vi "Find Item Locations by Path.vi"(5 "Insertion point if not found":bool, 6 "Only return first found":bool, 7 "Path":string, 8 "error in (no error)":errorcluster, 10 "Object Offset":i32, 11 "JSON":string) -> (0 "error out":errorcluster, 1 "Items":T1[](array[typedef]))   [LabVIEW 2017, in "JSONtext.lvlib"]
uses:
  JSONtext.lvlib
  Parsing/Found Items.ctl
  Parsing/Parsing State.ctl
  <vilib>/JDP Science/JDP Science Common Utilities/Trim Whitespace__JDP.vi
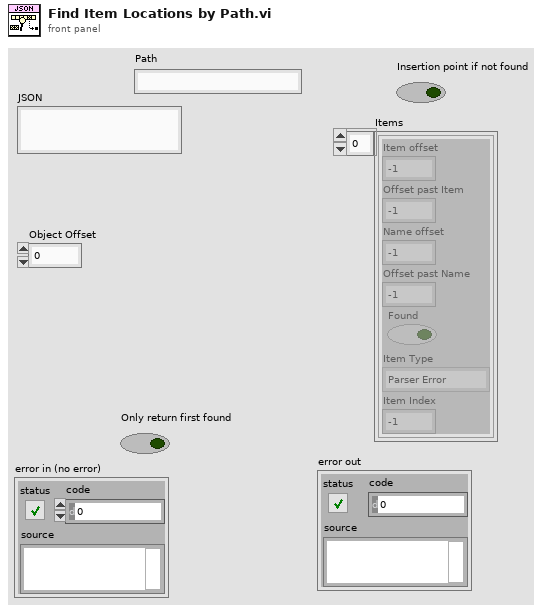
[diagram p1: front panel]
types:
  T1 = typedef "JSONtext.lvlib/Found Items.ctl" = cluster{"Item offset":i32, "Offset past Item":i32, "Name offset":i32, "Offset past Name":i32, "Found":bool, "Item Type":T2, "Item Index":i32}
  T2 = typedef "JSONtext.lvlib/Parsing State.ctl" = enum16{"Parser Error", "Object", "Array", "String", "Number/Other", "Leading Whitespace", "Object end", "Array end", "Value end"}
  T3 = cluster{"Type":T2, "Value start":i32, "Offset":i32}[]
  T4 = cluster{"Type":T2, "Value start":i32, "Offset":i32}
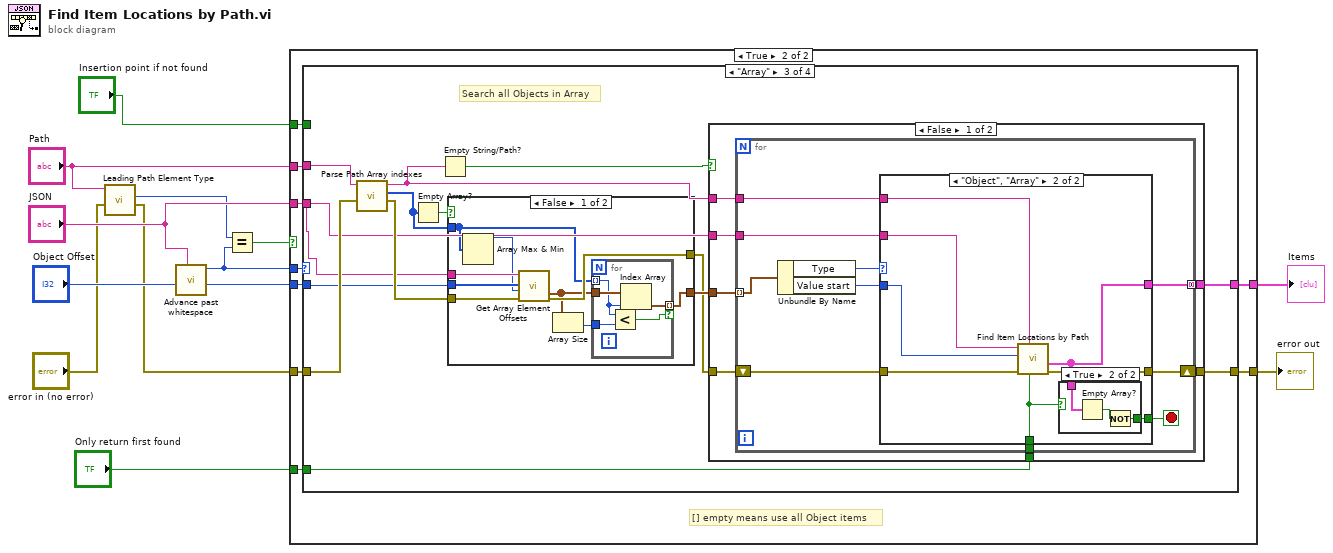
[diagram p0: block diagram]
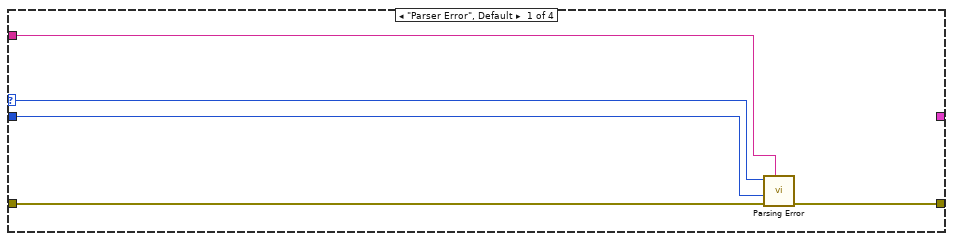
[diagram p3: hidden frame]
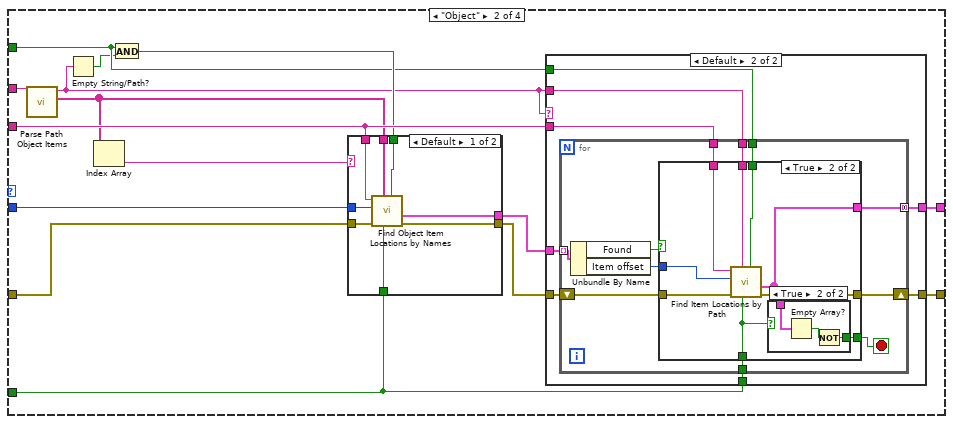
[diagram p4: hidden frame]
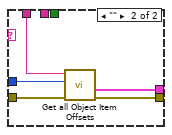
[diagram p5: hidden frame]
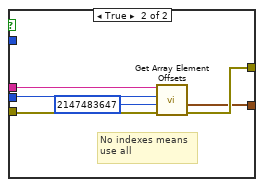
[diagram p9: hidden frame]
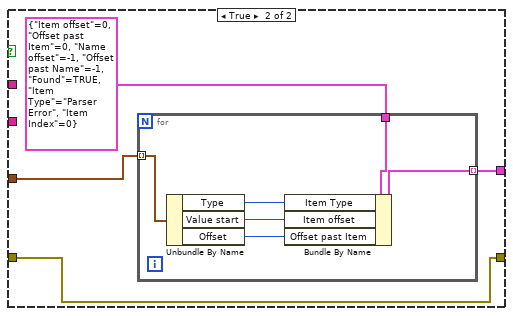
[diagram p12: hidden frame]
diagram:
  n1 = call "Leading Path Element Type.vi"("error in (no error)"="error in (no error)", "Path"="Path") -> ("error out"=w4:errorcluster, "Path Element Type"=w2:T2)  [unwired: 8 in]
  n2 = call "Advance past whitespace.vi"("JSON"="JSON", "Offset"="Object Offset") -> ("Offset of first non-whitespace"=w10:i32, "Parser State"=w3:T2)  [unwired: 8 in]
  n3 = Equal?(x=w2, y=w3) -> (x = y?=w1:bool)
  n4 = case shown="True" w1 {
    tunnel: [_ w23] -> w12
    tunnel: "JSON" -> [_ w15]
    tunnel: w10 -> [_ w16]
    tunnel: [w14 w22] -> w9
    tunnel: "Only return first found" -> [_ w21]
    tunnel: "Insertion point if not found" -> [_ w20]
    tunnel: "Path" -> [_ w19]
    tunnel: w4 -> [w14 w18]
    tunnel: w3 -> [_ w17]
    frame False {
    }
    frame True {
      # "[] empty means use all Object items"
      n5 = case shown="\"Array\"" w17 {
        selector: w17 -> [w26 _ _ _]
        tunnel: [_ w42 w103 _] -> w23
        tunnel: w18 -> [w28 w40 w100 w164]
        tunnel: [w27 w43 w104 w164] -> w22
        tunnel: w19 -> [_ w39 w101 _]
        tunnel: w21 -> [_ w33 w102 _]
        tunnel: w20 -> [_ w31 _ _]
        tunnel: w16 -> [w25 w38 w93 _]
        tunnel: w15 -> [w24 w41 w92 _]
        frame "Parser Error", Default {
          n6 = call "Parsing Error.vi"("JSON"=w24, "error in (no error)"=w28, "Offset past match"=w25, "State"=w26) -> ("error out"=w27:errorcluster)  [unwired: 7 in]
        }
        frame "Object" {
          n7 = call "Parse Path Object Items.vi"("Path with leading Object element"=w39) -> ("<JSON>items names"=w35:string[], "Rest or Path"=w29:string)  [unwired: 8 in, 1 out]
          n8 = Empty String/Path?(string/path=w29) -> (empty?=w30:bool)
          n9 = Index Array(array=w35) -> (element=w34:string)  [unwired: 1 in]
          n10 = And(x=w31, y=w30) -> (x .and. y?=w32:bool)
          n11 = case shown="Default" w34 {
            tunnel: w41 -> [w51 w56]
            tunnel: w40 -> [w50 w54]
            tunnel: w38 -> [w49 w55]
            tunnel: w35 -> [w48 _]
            tunnel: [w47 w53] -> w37
            tunnel: [w46 w52] -> w36
            tunnel: w33 -> [w45 _]
            tunnel: w32 -> [w44 _]
            frame Default {
              n12 = call "Find Object Item Locations by Names.vi"("Insertion point if not found"=w44, "Only return first found"=w45, "Item Names <JSON>"=w48, "error in (no error)"=w50, "Object Offset"=w49, "JSON"=w51) -> ("error out"=w47:errorcluster, "Items"=w46:T1[])  [unwired: 4 in]
            }
            frame "" {
              n13 = call "Get all Object Item Offsets.vi"("error in (no error)"=w54, "Offset"=w55, "JSON"=w56) -> ("error out"=w53:errorcluster, "Items"=w52:T1[])  [unwired: 6 in, 1 out]
            }
          }
          n14 = case shown="Default" w29 {
            tunnel: [w57 w66] -> w43
            tunnel: [w58 w65] -> w42
            tunnel: w41 -> [_ w64]
            tunnel: w29 -> [_ w63]
            tunnel: w37 -> [w57 w62]
            tunnel: w36 -> [w58 w61]
            tunnel: w33 -> [_ w60]
            tunnel: w31 -> [_ w59]
            frame "" {
            }
            frame Default {
              n15 = for {
                tunnel: [w76] -> w65 mode=concatenating
                tunnel: w64 -> [w75]
                tunnel: w63 -> [w74]
                tunnel: w61 -> [w72] mode=indexing
                shift-right: [w77] -> w66
                shift-left: w62 -> [w73]
                tunnel: w60 -> [w69]
                tunnel: w59 -> [w67]
                stop <- w68 stop-if-true
                n16 = Unbundle By Name(w72) -> ("Found"=w71:bool, "Item offset"=w70:i32)
                n17 = case shown="True" w71 {
                  tunnel: [w78 w87] -> w77
                  tunnel: [_ w81] -> w76
                  tunnel: w75 -> [_ w86]
                  tunnel: w74 -> [_ w85]
                  tunnel: w73 -> [w78 w84]
                  tunnel: w70 -> [_ w83]
                  tunnel: w69 -> [_ w82]
                  tunnel: [_ w80] -> w68
                  tunnel: w67 -> [_ w79]
                  frame False {
                  }
                  frame True {
                    n18 = call "Find Item Locations by Path.vi"("Insertion point if not found"=w79, "Only return first found"=w82, "Path"=w85, "error in (no error)"=w84, "Object Offset"=w83, "JSON"=w86) -> ("error out"=w87:errorcluster, "Items"=w81:T1[])  [unwired: 4 in]
                    n19 = case shown="True" w82 {
                      tunnel: w81 -> [_ w90]
                      tunnel: [_ w88] -> w80
                      frame False {
                      }
                      frame True {
                        n20 = Empty Array?(array=w90) -> (empty?=w89:bool)
                        n21 = Not(x=w89) -> (.not. x?=w88:bool)
                      }
                    }
                  }
                }
              }
            }
          }
        }
        frame "Array" {
          # "Search all Objects in Array"
          n22 = call "Parse Path Array indexes.vi"("error in (no error)"=w100, "Path with leading Array element"=w101) -> ("error out"=w94:errorcluster, "Indexes (empty means use all)"=w95:i32[], "Rest or Path"=w99:string)  [unwired: 7 in]
          n23 = Empty Array?(array=w95) -> (empty?=w97:bool)
          n24 = Empty String/Path?(string/path=w99) -> (empty?=w98:bool)
          n25 = case shown="False" w97 {
            tunnel: [w113 w120] -> w96
            tunnel: w95 -> [w106 _]
            tunnel: w94 -> [w111 w122]
            tunnel: w93 -> [w110 w123]
            tunnel: w92 -> [w109 w124]
            tunnel: [w108 w121] -> w91
            frame False {
              n26 = Array Max & Min(array=w106) -> (max value=w105:i32)  [unwired: 3 out]
              n27 = call "Get Array Element Offsets.vi"("error in (no error)"=w111, "Max Index"=w105, "Offset"=w110, "JSON"=w109) -> ("error out"=w108:errorcluster, "Elements"=w107:T3)  [unwired: 5 in, 1 out]
              n28 = Array Size(array=w107) -> (size(s)=w112:i32)
              n29 = for {
                tunnel: w106 -> [w116] mode=indexing
                tunnel: w107 -> [w118]
                tunnel: [w117] -> w113 mode=indexing if=w114
                tunnel: w112 -> [w115]
                n30 = Less?(x=w116, y=w115) -> (x < y?=w114:bool)
                n31 = Index Array(array=w118, index=w116) -> (element=w117:T4)
              }
            }
            frame True {
              # "No indexes means\nuse all"
              n32 = call "Get Array Element Offsets.vi"("error in (no error)"=w122, "Max Index"=2147483647, "Offset"=w123, "JSON"=w124) -> ("error out"=w121:errorcluster, "Elements"=w120:T3)  [unwired: 5 in, 1 out]
            }
          }
          n33 = case shown="False" w98 {
            tunnel: [w131 w154] -> w104
            tunnel: [w130 w155] -> w103
            tunnel: w96 -> [w129 w157]
            tunnel: w91 -> [w128 w154]
            tunnel: w92 -> [w127 _]
            tunnel: w102 -> [w126 _]
            tunnel: w99 -> [w125 _]
            frame False {
              n34 = for {
                tunnel: [w139] -> w130 mode=concatenating
                shift-right: [w140] -> w131
                shift-left: w128 -> [w141]
                tunnel: w125 -> [w138]
                tunnel: w129 -> [w137] mode=indexing
                tunnel: w127 -> [w135]
                tunnel: w126 -> [w133]
                stop <- w132 stop-if-true
                n35 = Unbundle By Name(w137) -> ("Type"=w136:T2, "Value start"=w134:i32)
                n36 = case shown="\"Object\", \"Array\"" w136 {
                  tunnel: w141 -> [w142 w150]
                  tunnel: [w142 w149] -> w140
                  tunnel: [_ w145] -> w139
                  tunnel: w138 -> [_ w148]
                  tunnel: w135 -> [_ w147]
                  tunnel: w134 -> [_ w146]
                  tunnel: w133 -> [_ w143]
                  tunnel: [_ w144] -> w132
                  frame "Parser Error", Default {
                  }
                  frame "Object", "Array" {
                    n37 = call "Find Item Locations by Path.vi"("Only return first found"=w143, "Path"=w148, "error in (no error)"=w150, "Object Offset"=w146, "JSON"=w147) -> ("error out"=w149:errorcluster, "Items"=w145:T1[])  [unwired: 5 in]
                    n38 = case shown="True" w143 {
                      tunnel: w145 -> [_ w153]
                      tunnel: [_ w151] -> w144
                      frame False {
                      }
                      frame True {
                        n39 = Empty Array?(array=w153) -> (empty?=w152:bool)
                        n40 = Not(x=w152) -> (.not. x?=w151:bool)
                      }
                    }
                  }
                }
              }
            }
            frame True {
              n41 = for {
                tunnel: w157 -> [w163] mode=indexing
                tunnel: T1 {"Item offset"=0, "Offset past Item"=0, "Name offset"=-1, "Offset past Name"=-1, "Found"=TRUE, "Item Type"=enum."Parser Error", "Item Index"=0} -> [w162]
                tunnel: [w161] -> w155 mode=indexing
                n42 = Unbundle By Name(w163) -> ("Type"=w158:T2, "Value start"=w159:i32, "Offset"=w160:i32)
                n43 = Bundle By Name(cluster=w162, "Item Type"=w158, "Item offset"=w159, "Offset past Item"=w160) -> (w161:T1)
              }
            }
          }
        }
        frame "String", "Number/Other" {
          # "Not an object or Array so Path ends here\n\n--> throw error?"
        }
      }
    }
  }
  "Items" <- w12
  "error out" <- w9
